vi "Example - Basic IPS-Init.vi"(0 "Connection Details":T4={"VISA resource name"="", "Comms Layer"=enum."Ethernet TCP/IP", "IP Address"="", "Serial Configuration"={"Baud Rate"=115200, "Parity"=0, "Data Bits"=8, "Stop Bits"=10, "Flow Control"=0}, "ISOBUS address"=-1} {"Serial Configuration"."Flow Control" items=["None", "XON/XOFF", "RTS/CTS", "XON/XOFF & RTS/CTS", "DTR/DSR", "XON/XOFF & DTR/DSR"]; "Serial Configuration"."Stop Bits" items=["1.0"=10, "2.0"=20]; "Serial Configuration"."Data Bits" items=["7"=7, "8"=8]; "Serial Configuration"."Parity" items=["None", "Odd", "Even"]; "Serial Configuration"."Baud Rate" items=["300"=300, "600"=600, "1200"=1200, "2400"=2400, "4800"=4800, "9600"=9600, "14400"=14400, "19200"=19200, "38400"=38400, "57600"=57600, "115200"=115200]}, 1 "Switch Present":string, 5 "Axis Group":string(combo)="GRPZ", 7 "ID Query (True)":bool, 9 "Clear Previous Connections (False)":bool, 11 "error in (no error)":errorcluster) -> (2 "Device Details":T6, 3 "Merc_Ref_LVL":T8, 4 "Merc_Ref_Mag":T8, 6 "Merc_Ref_MB1.T1":T8, 8 "Temp_Present?":bool, 10 "LVL_Present?":bool, 12 "ISOBUS address":T3=-1, 13 "Range_Data":T7 {"Current/Field (A/T)" format="%#.4f"}, 14 "Out Config 2":T5="PARA" caption="Output Configuration", 15 "error out":errorcluster)   [LabVIEW 2016, in "Mercury iXX.lvlib"]
uses:
  Mercury iXX.lvlib
  Public/Controls/Comms Transport Layer.ctl
  Public/Controls/Serial Settings.ctl
  Public/Controls/ISOBus Address.ctl
  Public/Libraries/Magnet/Controls/Output Configuration.ctl
  Public/Controls/Mercury Reference.ctl
  Private/Controls/Query Dynamic Reference.ctl
  Public/Libraries/System/Open/Open System.vi
  Public/Libraries/System/Read/Catalogue (Read).vi
  Public/Libraries/System/Read/DateTime (Read).vi
  Public/Libraries/Level Meter/Open/Open Level Meter Device.vi
  Public/Libraries/Temperature/Open/Open Temperature Device.vi
  Public/Libraries/Magnet/Open/Open Magnet Device.vi
  Public/Libraries/Magnet/Configuration/Read/Output Configuration (Read).vi
  Public/Libraries/Magnet/Configuration/Read/Current to Field Factor (Read).vi
  Public/Libraries/Magnet/Configuration/Set/Switch Present (Set).vi
  Public/Libraries/System.lvlib
  Public/Libraries/Level Meter.lvlib
  Public/Libraries/Magnet.lvlib
  Public/Libraries/Temperature.lvlib
panel:
  in  "Tab Control":enum32{"Connection", "Panel", "Error"}(tab)
  out "Number of Mag Units\nin the group":dbl
  out "Sys_time_stamp":timestamp
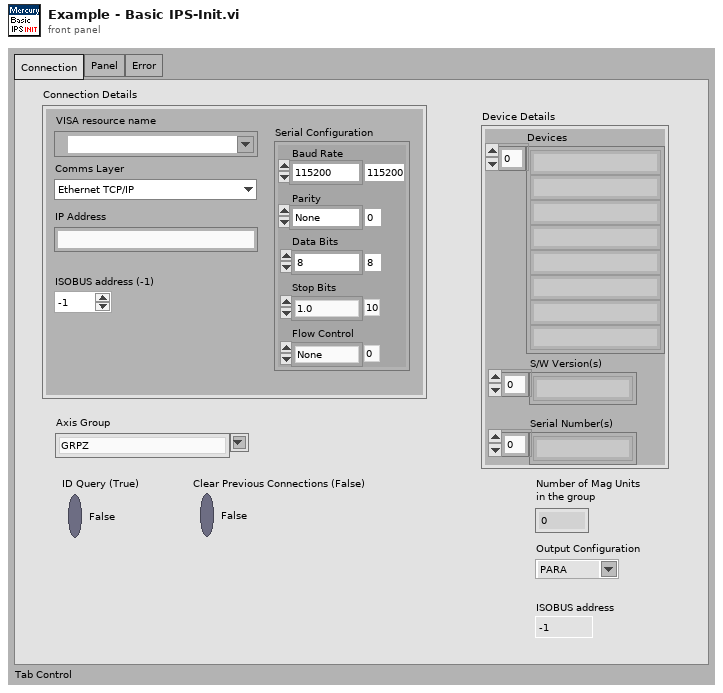
[diagram p1: front panel]
types:
  T1 = typedef "Mercury iXX.lvlib/Comms Transport Layer.ctl" = enum16{"Ethernet TCP/IP", "USB", "ISOBus - RS-232", "GPIB"}
  T2 = typedef "Mercury iXX.lvlib/Serial Settings.ctl" = cluster{"Baud Rate":u32, "Parity":u16, "Data Bits":u16, "Stop Bits":u16, "Flow Control":u16}
  T3 = typedef "Mercury iXX.lvlib/ISOBus Address.ctl" = i32
  T4 = cluster{"VISA resource name":refnum<visa-resource-name>, "Comms Layer":T1, "IP Address":string, "Serial Configuration":T2, "ISOBUS address":T3}
  T5 = typedef "Mercury iXX.lvlib/Magnet.lvlib/Output Configuration.ctl" = string
  T6 = cluster{"Devices":string[], "S/W Version(s)":string[], "Serial Number(s)":string[]}
  T7 = cluster{"Current/Field (A/T)":dbl, "Meter_V_Lim":dbl, "Meter_I_lim":dbl}
  T8 = typedef "Mercury iXX.lvlib/Mercury Reference.ctl" = cluster{"Comms":refnum<visa-resource-name>, "Device ID":string[], "Comms Layer":T1, "Command":string, "Query reference":T9}
  T9 = typedef "Mercury iXX.lvlib/Query Dynamic Reference.ctl" = refnum<vi>
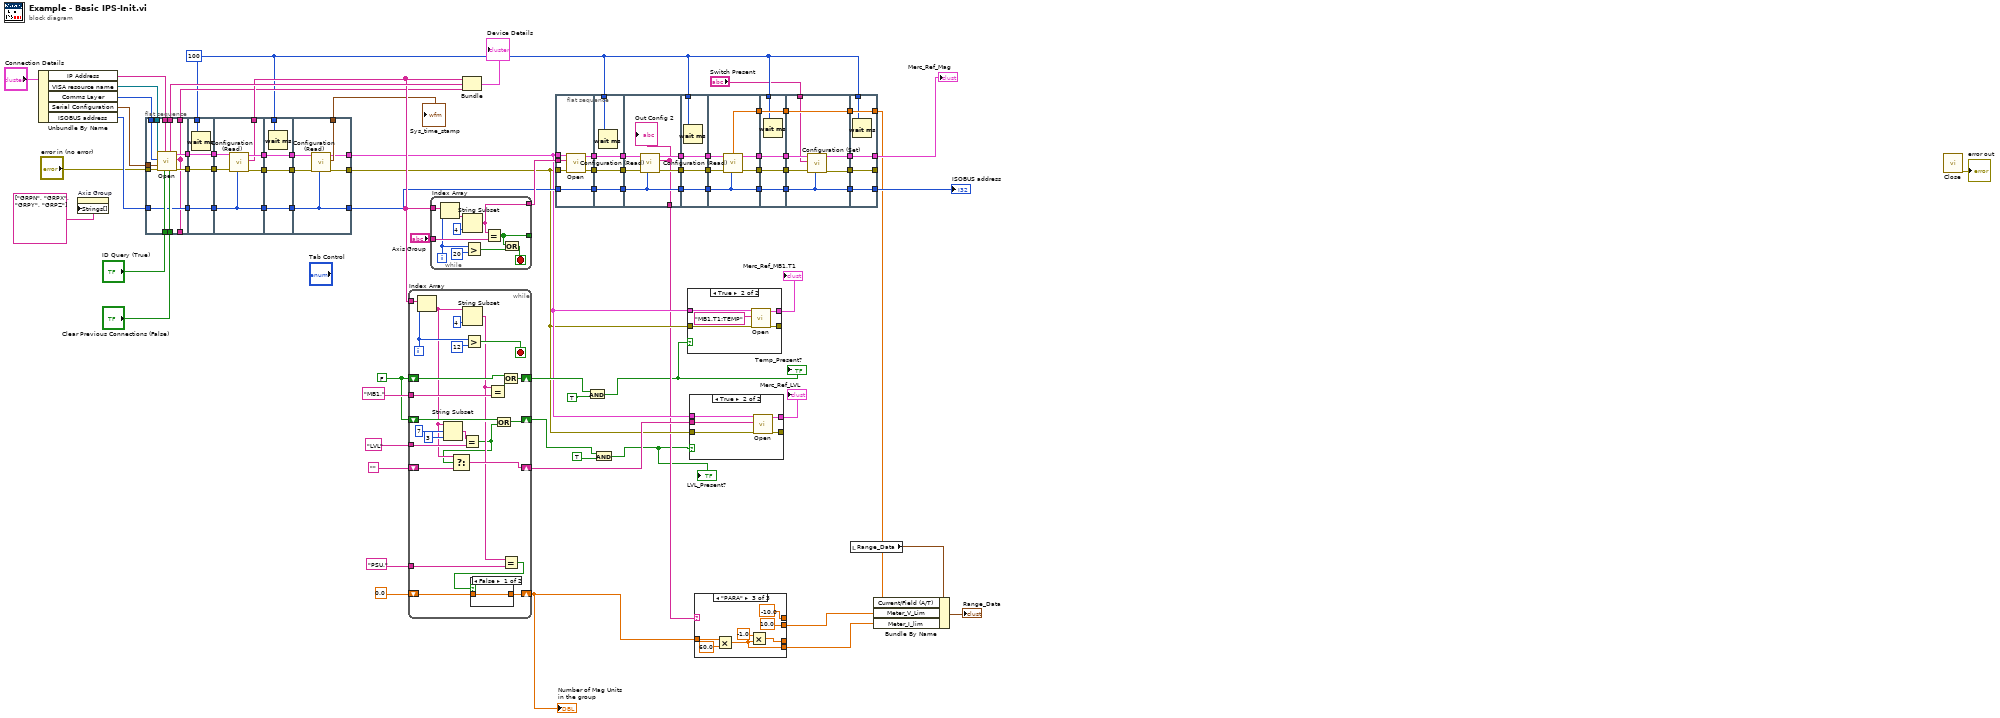
[diagram p0: block diagram]
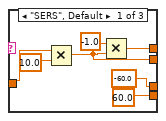
[diagram p4: hidden frame]
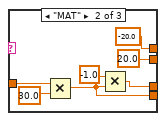
[diagram p5: hidden frame]
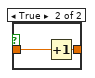
[diagram p6: hidden frame]
diagram:
  w2 = i16 100 ("Interval between messages (ms)")
  w55 = FALSE
  n1 = Unbundle By Name("Connection Details") -> ("IP Address"=w72:string, "VISA resource name"=w71:refnum<visa-resource-name>, "Comms Layer"=w70:T1, "Serial Configuration"=w73:T2, "ISOBUS address"=w62:T3)
  n2 = property on="Axis Group" class="CmbBox"("Strings[]"=string[] ["GRPN", "GRPX", "GRPY", "GRPZ"]) -> ()  [unwired: 2 in, 2 out]
  n3 = flat-sequence {
    tunnel: "error in (no error)" -> [w95]
    tunnel: "ID Query (True)" -> [w94]
    tunnel: "Clear Previous Connections (False)" -> [w93]
    tunnel: w73 -> [w90]
    tunnel: w72 -> [w89]
    tunnel: w71 -> [w88]
    tunnel: w70 -> [w87]
    tunnel: [w86] -> w69
    tunnel: [w92] -> w66
    tunnel: [w91] -> w65
    tunnel: w62 -> [w85]
    tunnel: [w85] -> w61
    tunnel: [w84] -> w12
    tunnel: [w84] -> _
    tunnel: w66 -> [w99]
    tunnel: w65 -> [w98]
    tunnel: [w99] -> w64
    tunnel: [w98] -> w63
    tunnel: w61 -> [w97]
    tunnel: [w97] -> w60
    tunnel: w2 -> [w96]
    tunnel: w64 -> [w104]
    tunnel: w63 -> [w103]
    tunnel: w60 -> [w105]
    tunnel: [w105] -> w59
    tunnel: [w102] -> w58
    tunnel: [w101] -> w57
    tunnel: [w100] -> w48
    tunnel: w59 -> [w109]
    tunnel: w58 -> [w108]
    tunnel: w57 -> [w107]
    tunnel: w2 -> [w106]
    tunnel: [w109] -> w51
    tunnel: [w108] -> w50
    tunnel: [w107] -> w49
    tunnel: w51 -> [w113]
    tunnel: w50 -> [w114]
    tunnel: w49 -> [w115]
    tunnel: [w112] -> w44
    tunnel: [w113] -> w47
    tunnel: [w111] -> w46
    tunnel: [w110] -> w45
    frame #0 {
      n4 = call-poly "Open.vi"("Clear Previous Connections (False)"=w93, "ID Query (True)"=w94, "IP Address"=w89, "error in (no error)"=w95, "Serial Configuration"=w90, "Comms Layer"=w87, "VISA resource name"=w88) -> ("error out"=w91:errorcluster, "Serial Number(s)"=w84:string[], "Mercury Reference Out"=w92:T8, "S/W Version(s)"=w86:string[])  [unwired: 1 out]
    }
    frame #1 {
      n5 = Wait (ms)(milliseconds to wait=w96) -> ()  [unwired: 1 out]
    }
    frame #2 {
      n6 = call-poly "Configuration (Read).vi"("ISOBUS address"=w105, "error in"=w103, "Mercury Reference In"=w104) -> ("error out"=w102:errorcluster, "Devices"=w100:string[], "Mercury Reference Out"=w101:T8)  [unwired: 6 out]
    }
    frame #3 {
      n7 = Wait (ms)(milliseconds to wait=w106) -> ()  [unwired: 1 out]
    }
    frame #4 {
      n8 = call-poly "Configuration (Read).vi"("ISOBUS address"=w113, "error in"=w114, "Mercury Reference In"=w115) -> ("error out"=w110:errorcluster, "time stamp"=w112:timestamp, "Mercury Reference Out"=w111:T8)  [unwired: 6 out]
    }
  }
  n9 = while {
    shift-right: [w136] -> w75
    shift-left: 0.0 -> [w135]
    tunnel: "PSU." -> [w132]
    tunnel: w48 -> [w131]
    shift-right: [w128] -> w67
    shift-left: w55 -> [w127]
    tunnel: "MB1." -> [w129]
    tunnel: "LVL" -> [w123]
    shift-right: [w121] -> w54
    shift-left: w55 -> [w122]
    shift-right: [w119] -> w52
    shift-left: "" -> [w120]
    i -> [w137]
    stop <- w133 stop-if-true
    n10 = Index Array(array=w131, index=w137) -> (element=w117:string)
    n11 = String Subset(string=w117, offset (0)=7, length (rest)=3 ("length (rest)")) -> (substring=w124:string)
    n12 = String Subset(string=w117, length (rest)=4 ("length (rest)")) -> (substring=w118:string)  [unwired: 1 out]
    n13 = Equal?(x=w124, y=w123) -> (x = y?=w116:bool)
    n14 = Select(t=w117, s=w116, f=w120) -> (s? t:f=w119:string)
    n15 = Greater?(x=w137, y=12) -> (0:w133:bool)
    n16 = Equal?(x=w118, y=w129) -> (x = y?=w130:bool)
    n17 = Or(x=w122, y=w116) -> (x .or. y?=w121:bool)
    n18 = Or(x=w127, y=w130) -> (x .or. y?=w128:bool)
    n19 = Equal?(x=w118, y=w132) -> (x = y?=w134:bool)
    n20 = case shown="False" w134 {
      tunnel: [w140 w142] -> w136
      tunnel: w135 -> [w140 w141]
      frame False {
      }
      frame True {
        n21 = Increment(x=w141) -> (x+1=w142:dbl)
      }
    }
  }
  "Number of Mag Units\nin the group" <- w75
  n22 = while {
    tunnel: w48 -> [w152]
    tunnel: [w143] -> w81
    tunnel: "Axis Group" -> [w149]
    tunnel: [w144] -> _
    i -> [w147]
    stop <- w146 stop-if-true
    n23 = Index Array(array=w152, index=w147) -> (element=w150:string)
    n24 = String Subset(string=w150, length (rest)=4 ("length (rest)")) -> (substring=w143:string)  [unwired: 1 out]
    n25 = Greater?(x=w147, y=20) -> (0:w145:bool)
    n26 = Equal?(x=w143, y=w149) -> (x = y?=w144:bool)
    n27 = Or(x=w144, y=w145) -> (x .or. y?=w146:bool)
  }
  n28 = Bundle("Devices"=w48, "S/W Version(s)"=w69, "Serial Number(s)"=w12) -> (→"Device Details":T6)  [unwired: 1 out]
  n29 = flat-sequence {
    tunnel: w81 -> [w158]
    tunnel: w45 -> [w155]
    tunnel: w46 -> [w154]
    tunnel: w47 -> [w153]
    tunnel: [w157] -> w42
    tunnel: [w156] -> w41
    tunnel: [w153] -> w40
    tunnel: w42 -> [w162]
    tunnel: w41 -> [w161]
    tunnel: w40 -> [w160]
    tunnel: [w162] -> w39
    tunnel: [w161] -> w38
    tunnel: [w160] -> w37
    tunnel: w2 -> [w159]
    tunnel: w39 -> [w168]
    tunnel: w38 -> [w167]
    tunnel: w37 -> [w166]
    tunnel: [w163] -> w25
    tunnel: [w166] -> w36
    tunnel: [w165] -> w35
    tunnel: [w164] -> w34
    tunnel: w36 -> [w172]
    tunnel: w35 -> [w171]
    tunnel: w34 -> [w170]
    tunnel: [w172] -> w33
    tunnel: [w171] -> w32
    tunnel: [w170] -> w31
    tunnel: w2 -> [w169]
    tunnel: w33 -> [w174]
    tunnel: w32 -> [w178]
    tunnel: w31 -> [w177]
    tunnel: [w174] -> w30
    tunnel: [w176] -> w29
    tunnel: [w175] -> w28
    tunnel: [w173] -> w27
    tunnel: w30 -> [w183]
    tunnel: w29 -> [w182]
    tunnel: w28 -> [w181]
    tunnel: w27 -> [w180]
    tunnel: w2 -> [w179]
    tunnel: [w183] -> w10
    tunnel: [w182] -> w9
    tunnel: [w181] -> w8
    tunnel: [w180] -> w7
    tunnel: w10 -> [w184]
    tunnel: w9 -> [w189]
    tunnel: w8 -> [w188]
    tunnel: w7 -> [w190]
    tunnel: [w184] -> w6
    tunnel: [w186] -> w5
    tunnel: [w185] -> w4
    tunnel: [w190] -> w3
    tunnel: "Switch Present" -> [w187]
    tunnel: [w192] -> w13
    tunnel: [w193] -> _
    tunnel: [w194] -> w24
    tunnel: [w195] -> w18
    tunnel: w6 -> [w195]
    tunnel: w5 -> [w194]
    tunnel: w4 -> [w193]
    tunnel: w3 -> [w192]
    tunnel: w2 -> [w191]
    frame #0 {
      n30 = call-poly "Open.vi"("error in (no error)"=w155, "Device Identifier"=w158, "Mercury Reference In"=w154) -> ("error out"=w156:errorcluster, "Mercury Reference Out"=w157:T8)  [unwired: 7 out]
    }
    frame #1 {
      n31 = Wait (ms)(milliseconds to wait=w159) -> ()  [unwired: 1 out]
    }
    frame #2 {
      n32 = call-poly "Configuration (Read).vi"("ISOBUS address"=w166, "error in"=w167, "Mercury Reference In"=w168) -> ("error out"=w164:errorcluster, "Out Config"=w163:T5, "Mercury Reference Out"=w165:T8)  [unwired: 6 out]
      "Out Config 2" <- w163
    }
    frame #3 {
      n33 = Wait (ms)(milliseconds to wait=w169) -> ()  [unwired: 1 out]
    }
    frame #4 {
      n34 = call-poly "Configuration (Read).vi"("ISOBUS address"=w174, "error in"=w177, "Mercury Reference In"=w178) -> ("error out"=w175:errorcluster, "AtoB"=w173:dbl, "Mercury Reference Out"=w176:T8)  [unwired: 6 out]
    }
    frame #5 {
      n35 = Wait (ms)(milliseconds to wait=w179) -> ()  [unwired: 1 out]
    }
    frame #6 {
      n36 = call-poly "Configuration (Set).vi"("ISOBUS address"=w184, "error in"=w188, "Switch Present"=w187, "Mercury Reference In"=w189) -> ("error out"=w185:errorcluster, "Mercury Reference Out"=w186:T8)  [unwired: 4 in, 2 out]
    }
    frame #7 {
      n37 = Wait (ms)(milliseconds to wait=w191) -> ()  [unwired: 1 out]
    }
  }
  n38 = And(x=w67, y=TRUE) -> (x .and. y?=w22:bool)
  "Temp_Present?" <- w22
  n39 = And(x=w54, y=TRUE) -> (x .and. y?=w21:bool)
  "LVL_Present?" <- w21
  n40 = case shown="True" w22 {
    tunnel: w45 -> [w196 w201]
    tunnel: w46 -> [w197 w200]
    tunnel: [w197 w199] -> w26
    tunnel: [w196 w198] -> _
    frame False {
    }
    frame True {
      n41 = call-poly "Open.vi"("error in (no error)"=w201, "Device Identifier"="MB1.T1:TEMP", "Mercury Reference In"=w200) -> ("error out"=w198:errorcluster, "Mercury Reference Out"=w199:T8)  [unwired: 7 out]
    }
  }
  "Merc_Ref_MB1.T1" <- w26
  n42 = case shown="True" w21 {
    tunnel: w45 -> [w203 w209]
    tunnel: w46 -> [w204 w208]
    tunnel: [w204 w207] -> w23
    tunnel: [w203 w206] -> _
    tunnel: w52 -> [_ w205]
    frame False {
    }
    frame True {
      n43 = call-poly "Open.vi"("error in (no error)"=w209, "Device Identifier"=w205, "Mercury Reference In"=w208) -> ("error out"=w206:errorcluster, "Mercury Reference Out"=w207:T8)  [unwired: 7 out]
    }
  }
  "Merc_Ref_LVL" <- w23
  n44 = case shown="\"PARA\"" w25 {
    tunnel: w75 -> [w214 w221 w230]
    tunnel: [60.0 ("y") w220 w227] -> w15
    tunnel: [-60.0 ("y") w219 w226] -> _
    tunnel: [w213 -20.0 ("y") -10.0 ("y")] -> _
    tunnel: [w212 20.0 ("y") 10.0 ("y")] -> w16
    frame "SERS", Default {
      n45 = Multiply(x=w214, y=10.0) -> (x*y=w212:dbl)
      n46 = Multiply(x=-1.0, y=w212) -> (x*y=w213:dbl)
    }
    frame "MAT" {
      n47 = Multiply(x=w221, y=30.0) -> (x*y=w220:dbl)
      n48 = Multiply(x=-1.0, y=w220) -> (x*y=w219:dbl)
    }
    frame "PARA" {
      n49 = Multiply(x=w230, y=60.0) -> (x*y=w227:dbl)
      n50 = Multiply(x=-1.0, y=w227) -> (x*y=w226:dbl)
    }
  }
  n51 = local read "Range_Data"() -> (w17:T7)
  n52 = Bundle By Name(cluster=w17, "Current/Field (A/T)"=w13, "Meter_V_Lim"=w16, "Meter_I_lim"=w15) -> (→"Range_Data":T7)
  n53 = call "Close.vi"() -> ("error out"=→"error out":errorcluster)  [unwired: 2 in, 9 out]
  "Sys_time_stamp" <- w44
  "Merc_Ref_Mag" <- w24
  "ISOBUS address" <- w18
